vi "APTmotorGet.vi"(0 "reference in":refnum<k7>[](array[refnum]), 3 "error in (no error)":errorcluster) -> (7 "reference out":refnum<k7>[](array[refnum]), 8 "Current position":sgl[](array[numeric]) min=0 max=500, 10 "error out":errorcluster)   [LabVIEW 2015]
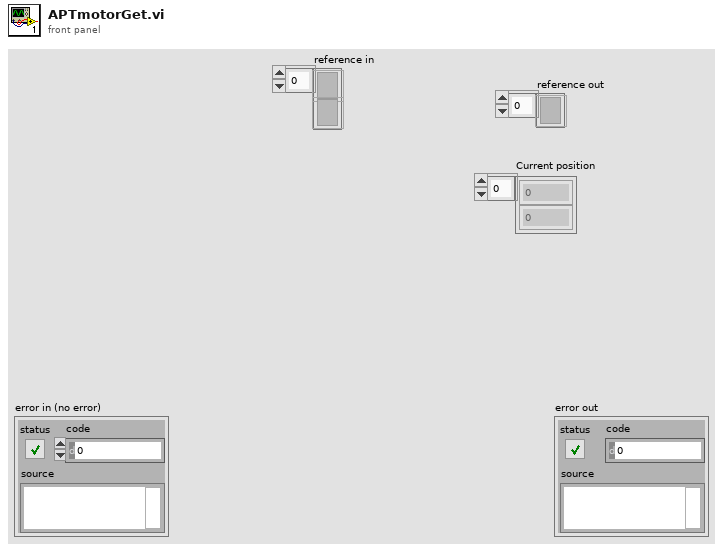
[diagram p1: front panel]
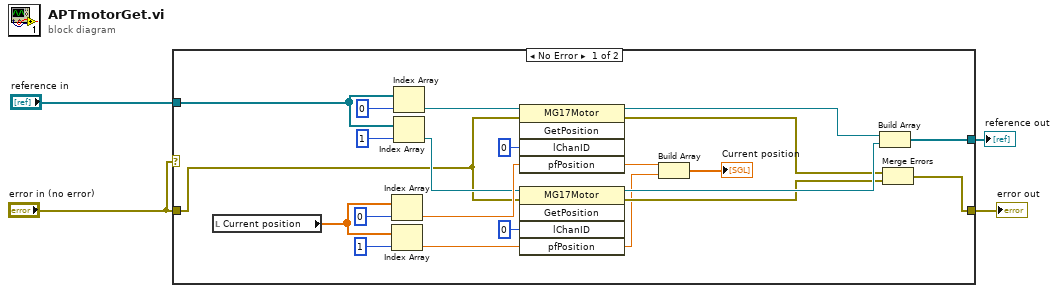
[diagram p0: block diagram]
diagram:
  n1 = case shown="No Error" "error in (no error)" {
    tunnel: [w15 w28] -> w4
    tunnel: "error in (no error)" -> [w16 w28]
    tunnel: [w14 w27] -> w2
    tunnel: "reference in" -> [w13 w27]
    frame No Error {
      n2 = local read "Current position"() -> (w5:sgl[])
      n3 = Index Array(array=w5, index=0) -> (element=w20:sgl)
      n4 = Index Array(array=w5, index=1) -> (element=w18:sgl)
      n5 = Index Array(array=w13, index=0) -> (element=w25:refnum<k7>)
      n6 = Index Array(array=w13, index=1) -> (element=w19:refnum<k7>)
      n7 = invoke class="MG17Motor" method="GetPosition"(reference=w25, error in=w16, "lChanID"=0, "pfPosition"=w20) -> (reference out=w9:refnum<k7>, error out=w10:errorcluster, "pfPosition"=w8:sgl)  [unwired: 1 in, 2 out]
      n8 = invoke class="MG17Motor" method="GetPosition"(reference=w19, error in=w16, "lChanID"=0, "pfPosition"=w18) -> (reference out=w12:refnum<k7>, error out=w11:errorcluster, "pfPosition"=w7:sgl)  [unwired: 1 in, 2 out]
      n9 = Build Array(w8, w7) -> (→"Current position":sgl[])
      n10 = Build Array(w9, w12) -> (w14:refnum<k7>[])
      n11 = Merge Errors(w10, w11) -> (w15:errorcluster)
    }
    frame Error {
    }
  }
  "error out" <- w4
  "reference out" <- w2
